vi "setpoint.vi"(7 "LWSR":refnum<class "Web Request.lvclass">, 10 "SP":dbl, 11 "ID":string) -> ()   [LabVIEW 2015]
uses:
  <vilib>/wsapi/Web Request.lvclass
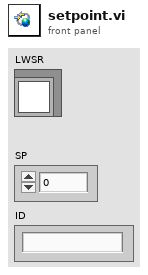
[diagram p1: front panel]
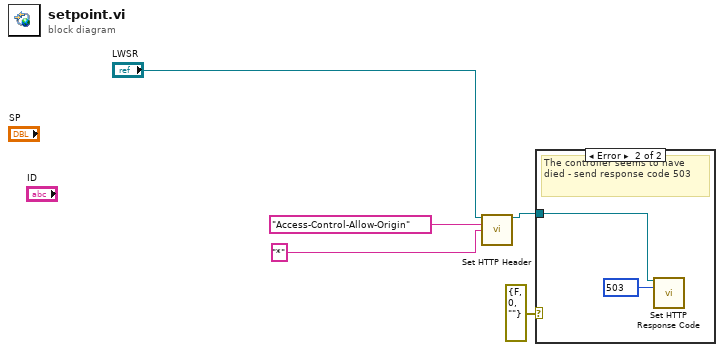
[diagram p0: block diagram]
diagram:
  n1 = call <vilib>:"Set HTTP Header.vi"("LabVIEW Web Service Request"="LWSR", "header"="Access-Control-Allow-Origin", "header value"="*") -> ("LabVIEW Web Service Request out"=w4:refnum<class "Web Request.lvclass">)  [unwired: 11 in, 1 out]
  n2 = case shown="Error" errorcluster {"status"=FALSE, "code"=0, "source"=""} ("error IO") {
    tunnel: w4 -> [_ w6]
    frame No Error {
    }
    frame Error {
      w7 = 503 items=["100"=100, "101"=101, "200"=200, "201"=201, "202"=202, "203"=203, "204"=204, "205"=205, "206"=206, "300"=300, "301"=301, "302"=302, "303"=303, "304"=304, "305"=305, "306"=306, "307"=307, "400"=400, "401"=401, "402"=402, "403"=403, "404"=404, "405"=405, "406"=406, "407"=407, "408"=408, "409"=409, "410"=410, "411"=411, "412"=412, "413"=413, "414"=414, "415"=415, "416"=416, "417"=417, "500"=500, "501"=501, "502"=502, "503"=503, "504"=504, "505"=505] ("response code (200)")
      # "The controller seems to have died - send response code 503"
      n3 = call <vilib>:"Set HTTP Response Code.vi"("LabVIEW Web Service Request"=w6, "response code (200)"=w7) -> ()  [unwired: 12 in, 2 out]
    }
  }
